vi "Initialize.vi"(6 "Source":tag, 8 "error in (no error)":errorcluster, 9 "Rate":dbl, 10 "Number Of Samples Per Channel":i32) -> (0 "error out":errorcluster, 3 "Digital Input out":refnum<class "Digital Input.lvclass">)   [LabVIEW 2021, in "Digital Input.lvlib" / "Digital Input.lvclass"]
uses:
  Digital Input.lvclass
  Digital Input.lvclass/Digital Input.ctl
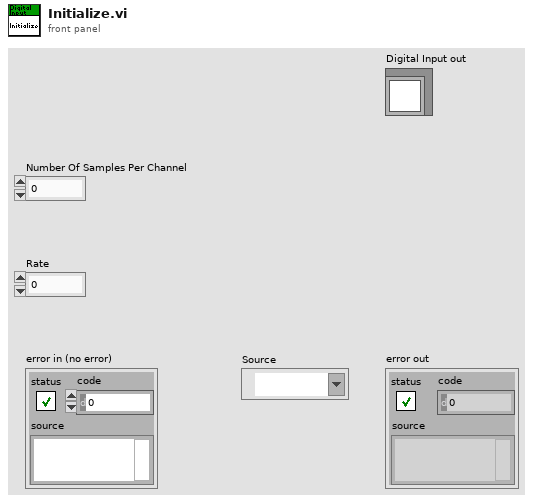
[diagram p1: front panel]
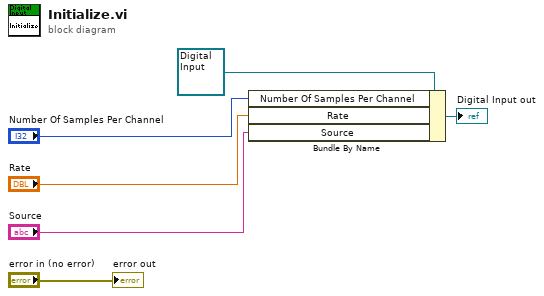
[diagram p0: block diagram]
diagram:
  n1 = Bundle By Name(cluster=refnum<class "Digital Input.lvclass"> refnum ("Digital Input in"), "Number Of Samples Per Channel"="Number Of Samples Per Channel", "Rate"="Rate", "Source"="Source") -> (→"Digital Input out":refnum<class "Digital Input.lvclass">)
  "error out" <- "error in (no error)"
